vi "StringBeginWith.vi"(10 "Begin With":string, 11 "String":string) -> (3 "StringBeginWith":bool)   [LabVIEW 2019]
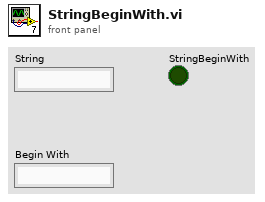
[diagram p1: front panel]
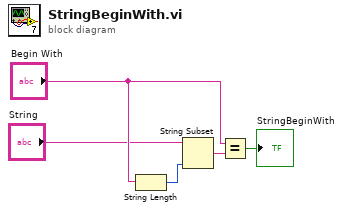
[diagram p0: block diagram]
diagram:
  n1 = String Length(string="Begin With") -> (length=w3:i32)
  n2 = String Subset(string="String", length (rest)=w3) -> (substring=w4:string)  [unwired: 1 in]
  n3 = Equal?(x="Begin With", y=w4) -> (x = y?=→"StringBeginWith":bool)
